vi "Condition Trigger.vi"(8 "Acquiring":bool, 9 "Pulse width (ticks)-Trial trig.":u32, 11 "Input signal":bool) -> (3 "Output signal":bool)   [LabVIEW 2020]
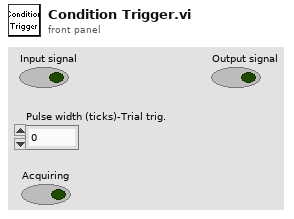
[diagram p1: front panel]
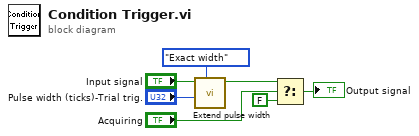
[diagram p0: block diagram]
diagram:
  n1 = call "Extend pulse width.vi"("Function"=enum16{"Minimum width", "Exact width"}."Exact width", "Pulse width (ticks)(80000=1ms @80MHz)"="Pulse width (ticks)-Trial trig.", "Input signal"="Input signal") -> ("Output signal"=w2:bool)  [unwired: 8 in]
  n2 = Select(t=w2, s="Acquiring", f=FALSE) -> (s? t:f=→"Output signal":bool)
